vi "plot_boat.vi"(0 "Desired Heading":dbl, 4 "Rudder Setpoint":T3 min=-0.95 max=0.95 scale=1.0..-1.0, 6 "Sail Setpoints":T4 {"MainSailSuggestion" min=0.0 max=1.0; "JibSailSuggestion" min=0.0 max=1.0}, 7 "Trace Path":bool=TRUE, 8 "Heading":dbl, 9 "MapDistanceInfo":T1 {"Top Left Pixel UTM"."North" format="%#_10f"; "Top Left Pixel UTM"."East" format="%#_8f"; "Bottom Right Pixel UTM"."North" format="%#_10f"; "Bottom Right Pixel UTM"."East" format="%#_8f"}, 10 "UTM Location":T2 {"North" format="%#_10f"; "East" format="%#_8f"}, 11 "Map in":T5) -> (1 "MapDistanceInfo OUT":T1 {"Top Left Pixel UTM"."North" format="%#_10f"; "Top Left Pixel UTM"."East" format="%#_8f"; "Bottom Right Pixel UTM"."North" format="%#_10f"; "Bottom Right Pixel UTM"."East" format="%#_8f"}, 2 "Boat Outside Img":bool, 3 "Map Out":T5)   [LabVIEW 2013]
uses:
  <vilib>/vision/Image Controls.llb/IMAQ Image.ctl
  cRIO_Code/Data/TypeDefs/UTM Location.ctl
  TypeDef/map_metadata.ctl
  cRIO_Code/Data/TypeDefs/Sail Set Suggestions.ctl
  cRIO_Code/Data/TypeDefs/Rudder Set Suggestions.ctl
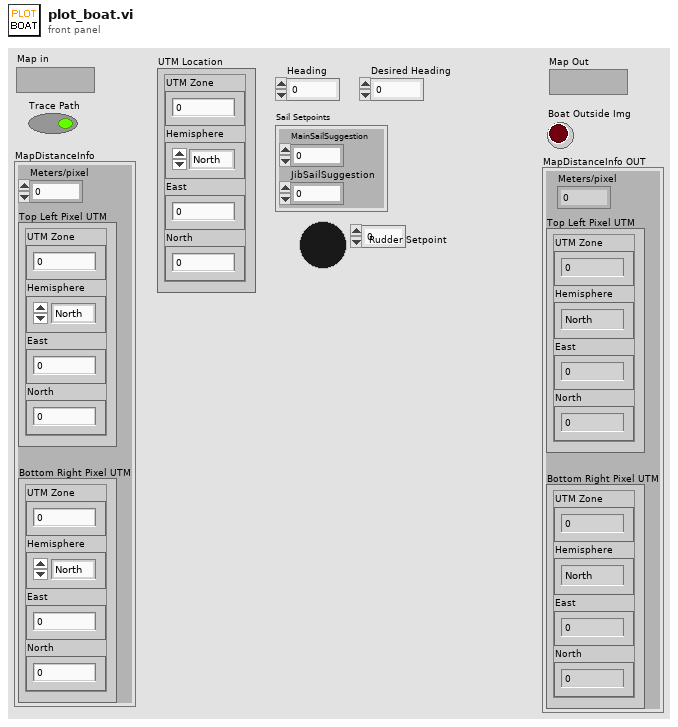
[diagram p1: front panel]
types:
  T1 = typedef "map_metadata.ctl" = cluster{"Meters/pixel":dbl, "Top Left Pixel UTM":T2, "Bottom Right Pixel UTM":T2}
  T2 = typedef "UTM Location.ctl" = cluster{"UTM Zone":dbl, "Hemisphere":enum16{"North", "South"}, "East":dbl, "North":dbl}
  T3 = typedef "Rudder Set Suggestions.ctl" = dbl
  T4 = typedef "Sail Set Suggestions.ctl" = cluster{"MainSailSuggestion":dbl, "JibSailSuggestion":dbl}
  T5 = typedef "IMAQ Image.ctl" = refnum<image>
  T6 = typedef "boat_overlay_references.ctl" = cluster{"Boat Icon, Unrotated":T5, "Boat Icon, Rotated":T5, "Mainsail Icon, Unrotated":T5, "Mainsail Icon, Rotated":T5, "Jib Icon, Rotated":T5, "Jib Icon, Unrotated":T5, "Rudder Icon, Rotated":T5, "Rudder Icon, Unrotated":T5}
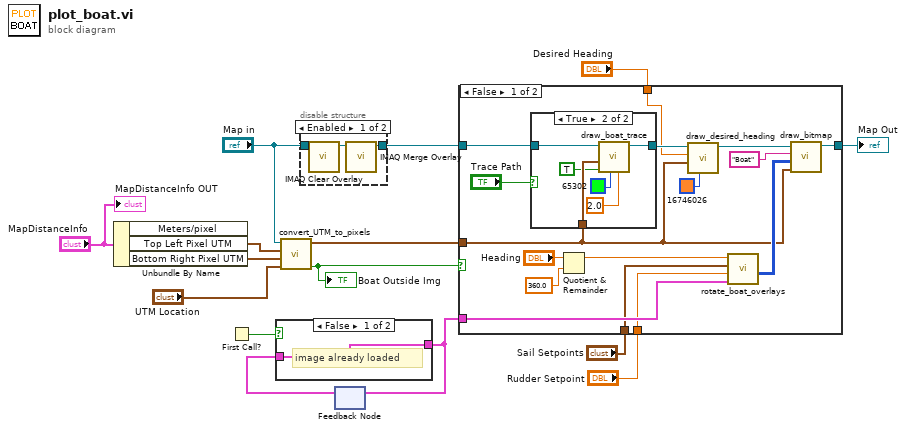
[diagram p0: block diagram]
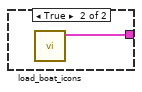
[diagram p5: hidden frame]
diagram:
  n1 = Unbundle By Name("MapDistanceInfo") -> ("Top Left Pixel UTM"=w7:T2, "Bottom Right Pixel UTM"=w6:T2)  [unwired: 1 out]
  n2 = First Call?() -> (First Call?: T/F=w3:bool)
  n3 = call "convert_UTM_to_pixels.vi"("UTM position of Boat"="UTM Location", "Bottom Right Pixel UTM"=w6, "Top Left Pixel UTM"=w7, "Map in"="Map in") -> ("Boat Outside Img"=w10:bool, "Position"=w9:cluster{"X":i32, "Y":i32})  [unwired: 6 in]
  "Boat Outside Img" <- w10
  n4 = disable-structure shown="Enabled" {
    disable-tunnel: [w17 w19] -> w14
    disable-tunnel: "Map in" -> [w16 w19]
    frame Enabled {
      n5 = call "IMAQ Clear Overlay"("Image"=w16) -> ("Image Out"=w18:T5)  [unwired: 2 in, 8 out]
      n6 = call "IMAQ Merge Overlay"("Image Src"=w18) -> ("Image Dst Out"=w17:T5)  [unwired: 4 in, 6 out]
    }
    frame Disabled {
    }
  }
  n7 = feedback #1() -> (w2:T6)  [unwired: 1 in]
  n8 = case shown="False" w3 {
    tunnel: [w20 w21] -> w15
    tunnel: w2 -> [w20 _]
    frame False {
      # "image already loaded"
    }
    frame True {
      n9 = call "load_boat_icons.vi"() -> ("Boat Overlay References Out"=w21:T6)  [unwired: 11 in]
    }
  }
  n10 = feedback-in #1(w15) -> ()
  n11 = case shown="False" w10 {
    tunnel: [w36 w45] -> w13
    tunnel: w14 -> [w35 w45]
    tunnel: w15 -> [w30 _]
    tunnel: w9 -> [w23 _]
    tunnel: "Sail Setpoints" -> [w29 _]
    tunnel: "Rudder Setpoint" -> [w28 _]
    tunnel: "Desired Heading" -> [w24 _]
    frame False {
      n12 = case shown="True" "Trace Path" {
        tunnel: [w38 w43] -> w26
        tunnel: w35 -> [w38 w42]
        tunnel: w23 -> [_ w41]
        frame False {
        }
        frame True {
          n13 = call "draw_boat_trace.vi"("Radius (px)"=2.0, "circle color"=u32 65302, "Merge Overlay?"=TRUE, "Position"=w41, "Image In"=w42) -> ("Image Out"=w43:T5)  [unwired: 6 in]
        }
      }
      n14 = Quotient & Remainder(x="Heading", y=360.0) -> (x-y*floor(x/y)=w33:dbl)  [unwired: 1 out]
      n15 = call "draw_desired_heading.vi"("circle color"=u32 16746026, "Boat Position"=w23, "Desired Heading"=w24, "Image In"=w26) -> ("Image Out"=w25:T5)  [unwired: 7 in]
      n16 = call "rotate_boat_overlays.vi"("Overlay References In"=w30, "Rudder Setpoint"=w28, "Sail Setpoints"=w29, "Heading"=w33) -> ("Rotated Boat Icon Bitmap Out"=w37:u32[][])  [unwired: 6 in, 1 out]
      n17 = call "draw_bitmap.vi"("Position"=w23, "Boat Bitmap"=w37, "Group"="Boat", "Image In"=w25) -> ("Image Out"=w36:T5)  [unwired: 3 out]
    }
    frame True {
      # "don't draw\nif boat\noutside\nimage why not? lol"
    }
  }
  "Map Out" <- w13
  "MapDistanceInfo OUT" <- "MapDistanceInfo"
